vi "Disconnect.vi"(8 "error in (no error)":errorcluster, 11 "3446X in":refnum<class "3446X.lvclass">) -> (0 "error out":errorcluster, 3 "3446X out":refnum<class "3446X.lvclass">)   [LabVIEW 2018, in "3446X.lvlib" / "3446X.lvclass"]
uses:
  3446X.lvclass
  3446X.lvclass/3446X.ctl
  <instrlib>/Agilent 3446X Series/Agilent 3446X Series.lvlib
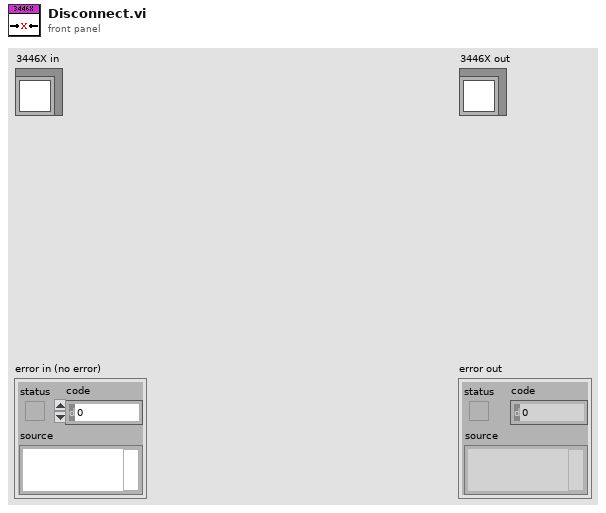
[diagram p1: front panel]
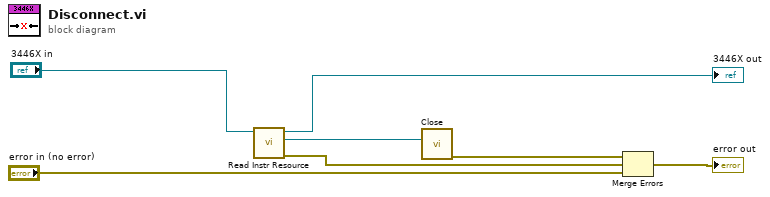
[diagram p0: block diagram]
diagram:
  n1 = call "Read Instr Resource.vi"("3446X in"="3446X in") -> ("error out"=w4:errorcluster, "Instr Resource"=w1:refnum<visa-resource-name>, "3446X out"=→"3446X out":refnum<class "3446X.lvclass">)  [unwired: 8 in]
  n2 = call <instrlib>:"Close.vi"("VISA resource name"=w1) -> ("error out"=w5:errorcluster)  [unwired: 10 in]
  n3 = Merge Errors(w5, w4, "error in (no error)") -> (→"error out":errorcluster)
